vi "EnCoder.vi"(6 "Reset Counter":bool, 8 "Encoder PPR":dbl=52.0, 9 "Gear Ratio":i32=30, 10 "R(mm)":dbl=30.0, 11 "error in":errorcluster) -> (1 "ENC Val. mm":T2, 2 "ENC":T1, 3 "error out":errorcluster)   [LabVIEW 2018]
uses:
  <vilib>/myRIO/Common/Instrument Driver Framework/myRIO v1.0/Encoder/typedefs/Encoder Count Direction Enum.ctl
  <vilib>/myRIO/Common/Instrument Driver Framework/myRIO v1.0/Encoder/typedefs/Encoder Signal Mode.ctl
  <vilib>/myRIO/Common/Instrument Driver Framework/myRIO v1.0/Encoder/typedefs/Encoder Channels Enum.ctl
  <vilib>/myRIO/Common/Instrument Driver Framework/Utilities/typedefs/Generic FPGA Reference.ctl
  <vilib>/myRIO/Common/Instrument Driver Framework/Utilities/typedefs/myRIO v1.0 Reference.ctl
  <vilib>/myRIO/Common/Instrument Driver Framework/Utilities/typedefs/Hardware Version Enum.ctl
  <vilib>/myRIO/Common/Instrument Driver Framework/Utilities/typedefs/myRIO Generic Hardware Reference.ctl
  <vilib>/myRIO/Instrument Drivers/Onboard IO/Encoder/typedefs/Encoder Reference.ctl
  <vilib>/myRIO/Instrument Drivers/Onboard IO/Encoder/Encoder.lvlib
  <vilib>/myRIO/Instrument Drivers/Onboard IO/Encoder/vis/Read.vi
  <vilib>/myRIO/Common/Instrument Driver Framework/myRIO v1.0/Encoder/typedefs/Encoder Configuration v1.0.ctl
  <vilib>/userdefined/High Color/nirio_resource_hc.ctl
  <vilib>/myRIO/Common/Instrument Driver Framework/myRIO v1.0/Encoder/vis/myRIO v1.1 Open Encoder.vi
  <vilib>/myRIO/Common/Instrument Driver Framework/myRIO v1.0/Encoder/vis/myRIO v1.0 Configure Encoder.vi
  <vilib>/myRIO/Instrument Drivers/Onboard IO/Encoder/vis/myRIO Encoder Open.xnode
  <vilib>/myRIO/Common/Instrument Driver Framework/Utilities/vis/Is FPGA Ref Available.vi
  <vilib>/myRIO/Express VI/Onboard IO/Encoder/Encoder Express VI.xnode
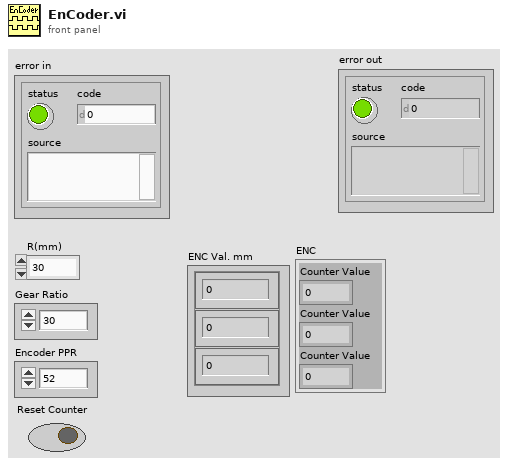
[diagram p1: front panel]
types:
  T1 = cluster{"Counter Value":i32, "Counter Value":i32, "Counter Value":i32}
  T2 = cluster{"Numeric Control":dbl, "Numeric Control":dbl, "Numeric Control":dbl}
  T3 = cluster{"Counter Value":dbl, "Counter Value":dbl, "Counter Value":dbl}
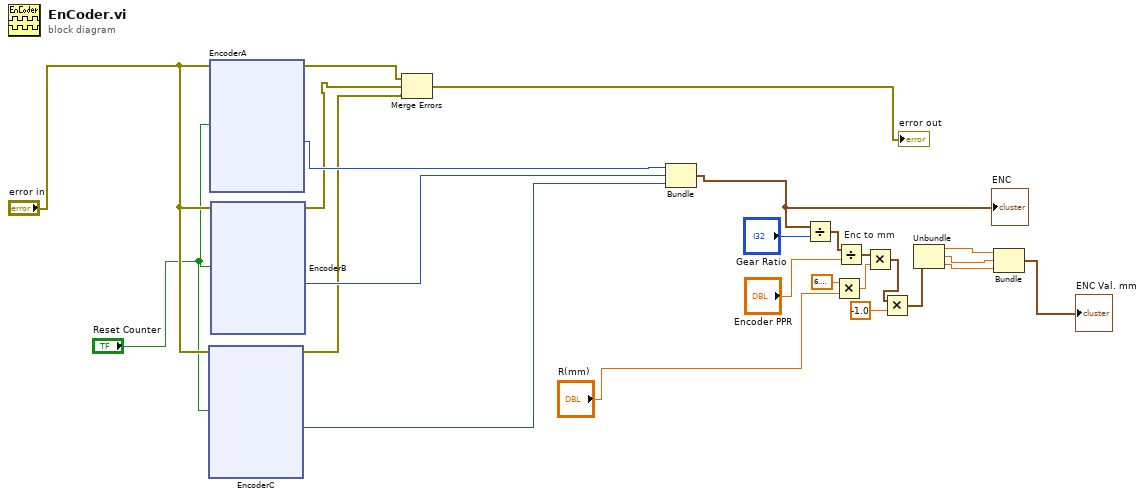
[diagram p0: block diagram]
diagram:
  n1 = xnode "EncoderC"("Reset Counter"="Reset Counter", "error in (no error)"="error in") -> ("Counter Value"=w14:i32, "error out"=w9:errorcluster)  [unwired: 2 out]
  n2 = xnode "EncoderA"("Reset Counter"="Reset Counter", "error in (no error)"="error in") -> ("Counter Value"=w13:i32, "error out"=w11:errorcluster)  [unwired: 2 out]
  n3 = xnode "EncoderB"("Reset Counter"="Reset Counter", "error in (no error)"="error in") -> ("Counter Value"=w15:i32, "error out"=w10:errorcluster)  [unwired: 2 out]
  n4 = Merge Errors(w11, w10, w9) -> (→"error out":errorcluster)
  n5 = Bundle("Counter Value"=w13, "Counter Value"=w15, "Counter Value"=w14) -> (w23:T1)  [unwired: 1 in]
  "ENC" <- w23
  n6 = Divide(x=w23, y="Gear Ratio") -> (x/y=w21:T3)
  n7 = Multiply(x=6.283185307179586, y="R(mm)") -> (x*y=w18:dbl)
  n8 = Divide(x=w21, y="Encoder PPR") -> (x/y=w19:T3)
  n9 = Multiply "Enc to mm"(x=w19, y=w18) -> (x*y=w2:T3)
  n10 = Multiply(x=w2, y=-1.0) -> (x*y=w1:T3)
  n11 = Unbundle(w1) -> ("Counter Value"=w4:dbl, "Counter Value"=w6:dbl, "Counter Value"=w5:dbl)
  n12 = Bundle("Counter Value"=w4, "Counter Value"=w6, "Counter Value"=w5) -> (→"ENC Val. mm":T3)  [unwired: 1 in]
